vi "Test Sine Wave Diogo.vi"() -> ()   [LabVIEW 2016]
uses:
  <vilib>/measure/NI_MABase.lvlib
panel:
  out "size(s)":i32
  out "Waveform Graph":waveform(dbl)(graph)
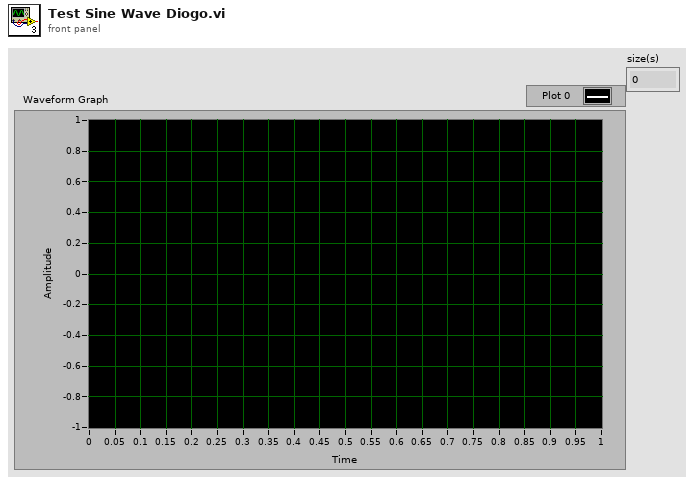
[diagram p1: front panel]
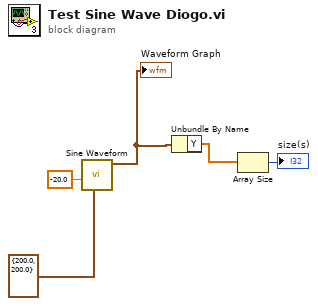
[diagram p0: block diagram]
diagram:
  n1 = call <vilib>:"Sine Waveform.vi"("sampling info"=cluster{"Fs":dbl, "#s":dbl} {"Fs"=200.0, "#s"=200.0}, "phase"=-20.0) -> ("signal out"=w3:waveform(dbl))  [unwired: 8 in, 1 out]
  "Waveform Graph" <- w3
  n2 = Unbundle By Name(w3) -> ("Y"=w2:dbl[])
  n3 = Array Size(array=w2) -> (size(s)=→"size(s)":i32)
